vi "Get Owning Path Default Value.vi"(0 "SA 26GHz Path Group in":refnum<class "SA 26GHz Path Group.lvclass">, 11 "error in":errorcluster) -> (4 "SA 26GHz Path Group out":refnum<class "SA 26GHz Path Group.lvclass">, 6 "Path":refnum<class "Path.lvclass">, 15 "error out":errorcluster)   [LabVIEW 2023, in "RFFixtureCharact.PXI.lvlib" / "SA 26GHz Path Group.lvclass"]
uses:
  SA 26GHz Path Group.lvclass
  SA 26GHz Path Group.lvclass/SA 26GHz Path Group.ctl
  Common/Base Classes/Path/Path.lvclass
  Paths/SA 26GHz Path/SA 26GHz Path.lvclass
  C:/srd-semi-rfcal-software - Main/AuxTools/STSRFFixtureCharactUtility/Source/Code Modules/Fixture/Public/Base Classes/Scalar/SA Path/SA Path.lvclass
  C:/srd-semi-rfcal-software - Main/AuxTools/STSRFFixtureCharactUtility/Source/Code Modules/Fixture/Public/Base Classes/Scalar/SA Abstract Path/SA Abstract Path.lvclass
  C:/srd-semi-rfcal-software - Main/AuxTools/STSRFFixtureCharactUtility/Source/Code Modules/Fixture/Public/Base Classes/Scalar/Scalar Path/Scalar Path.lvclass
  C:/srd-semi-rfcal-software - Main/AuxTools/STSRFFixtureCharactUtility/Source/Code Modules/Common/Base Classes/Path/Path.lvclass
  C:/srd-semi-rfcal-software - Main/AuxTools/STSRFFixtureCharactUtility/Source/Code Modules/Fixture/PXI/Scalar/Paths/SA 26GHz Path/SA 26GHz Path.lvclass
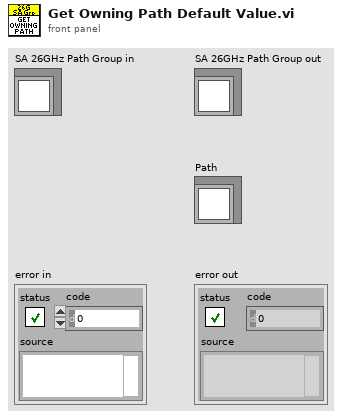
[diagram p1: front panel]
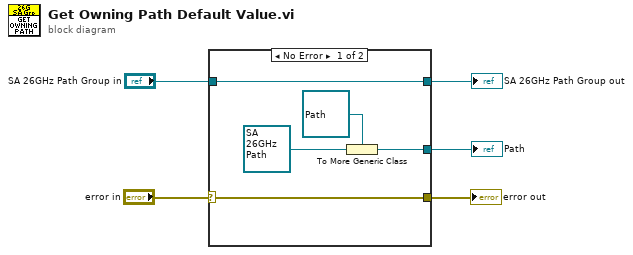
[diagram p0: block diagram]
diagram:
  n1 = case shown="No Error" "error in" {
    selector: "error in" -> [w10 w11]
    tunnel: [w8 _] -> w3
    tunnel: [w10 w11] -> w2
    tunnel: [w9 w12] -> w4
    tunnel: "SA 26GHz Path Group in" -> [w9 w12]
    frame No Error {
      n2 = To More Generic Class(target class=refnum<class "Path.lvclass"> refnum ("Path"), reference=refnum<class "SA 26GHz Path.lvclass"> refnum ("RFFixtureCharact.PXI.lvlib:SA 26GHz Path.lvclass")) -> (generic class reference=w8:refnum<class "Path.lvclass">)
    }
    frame Error {
    }
  }
  "error out" <- w2
  "SA 26GHz Path Group out" <- w4
  "Path" <- w3
